vi "User exists.vi"(8 "error in":errorcluster, 10 "user":string="perro", 11 "Array":T1[](array[typedef])) -> (0 "error out":errorcluster, 1 "Position":i32, 2 "User-data cluster":T1, 4 "exist?":bool)   [LabVIEW 2012]
uses:
  typedef/User_Data_Cluster.ctl
  typedef/User Accounts.ctl
panel:
  in  "User-datacluster":T1
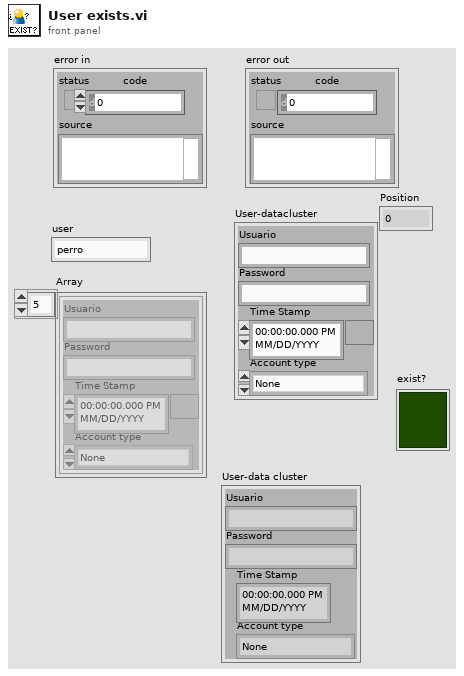
[diagram p1: front panel]
types:
  T1 = typedef "User_Data_Cluster.ctl" = cluster{"Usuario":string, "Password":string, "Account type":T2, "Time Stamp":timestamp}
  T2 = typedef "User Accounts.ctl" = enum16{"None", "User", "Admin"}
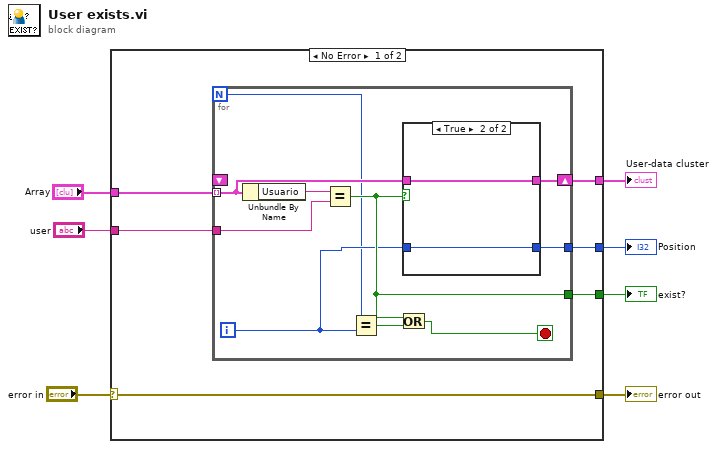
[diagram p0: block diagram]
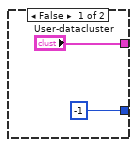
[diagram p2: hidden frame]
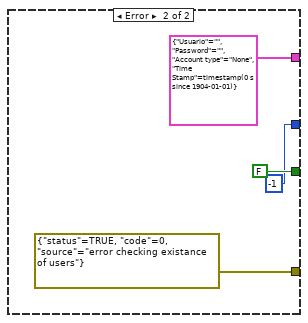
[diagram p3: hidden frame]
diagram:
  n1 = case shown="No Error" "error in" {
    selector: "error in" -> [w10 _]
    tunnel: [w13 T1 {"Usuario"="", "Password"="", "Account type"=enum."None", "Time Stamp"=timestamp(0 s since 1904-01-01)} ("User-data cluster")] -> w2
    tunnel: "Array" -> [w12 _]
    tunnel: [w11 FALSE] -> w6
    tunnel: [w10 errorcluster {"status"=TRUE, "code"=0, "source"="error checking existance of users"} ("error IO")] -> w5
    tunnel: "user" -> [w9 _]
    tunnel: [w8 -1] -> w1
    frame No Error {
      n2 = for {
        N -> [w14]
        tunnel: w12 -> [w21] mode=indexing
        shift-right: [w22] -> w13
        shift-left: _ -> [_]
        tunnel: [w19] -> w11
        tunnel: w9 -> [w18]
        tunnel: [w17] -> w8
        i -> [w15]
        stop <- w16 stop-if-true
        n3 = Unbundle By Name(w21) -> ("Usuario"=w23:string)
        n4 = Equal?(x=w23, y=w18) -> (x = y?=w19:bool)
        n5 = Equal?(x=w14, y=w15) -> (x = y?=w20:bool)
        n6 = Or(x=w19, y=w20) -> (x .or. y?=w16:bool)
        n7 = case shown="True" w19 {
          tunnel: w21 -> [_ w27]
          tunnel: ["User-datacluster" w27] -> w22
          tunnel: w15 -> [_ w26]
          tunnel: [-1 w26] -> w17
          frame False {
          }
          frame True {
          }
        }
      }
    }
    frame Error {
    }
  }
  "error out" <- w5
  "exist?" <- w6
  "User-data cluster" <- w2
  "Position" <- w1
